vi "CountStats.vi"() -> ()   [LabVIEW 2014]
uses:
  <instrlib>/Agilent 532XX Series/Public/Configure/Configure Channel (Basic).vi
  <instrlib>/Agilent 532XX Series/Public/Configure/Configure Channel (Voltage Range).vi
  <instrlib>/Agilent 532XX Series/Public/Configure/Configure Channel (Slop).vi
  <instrlib>/Agilent 532XX Series/Public/Configure/Configure Channel (Threshold Voltage).vi
  <instrlib>/Agilent 532XX Series/Public/Configure/Measurement/Configure Measurement (Totalize Timed).vi
  <instrlib>/Agilent 532XX Series/Public/Data/Read Measurement (Statistics).vi
  <instrlib>/Agilent 532XX Series/Agilent 532XX Series.lvlib
panel:
  in  "Sample Count (1)":i32=1
  out "Standard Deviation":dbl
  out "Maximum":dbl format="%#_12g"
  out "Minimum":dbl format="%#_12g"
  out "error out":errorcluster
  out "Measurement":dbl format="%#_12g"
  in  "VISA resource name":refnum<visa-resource-name>
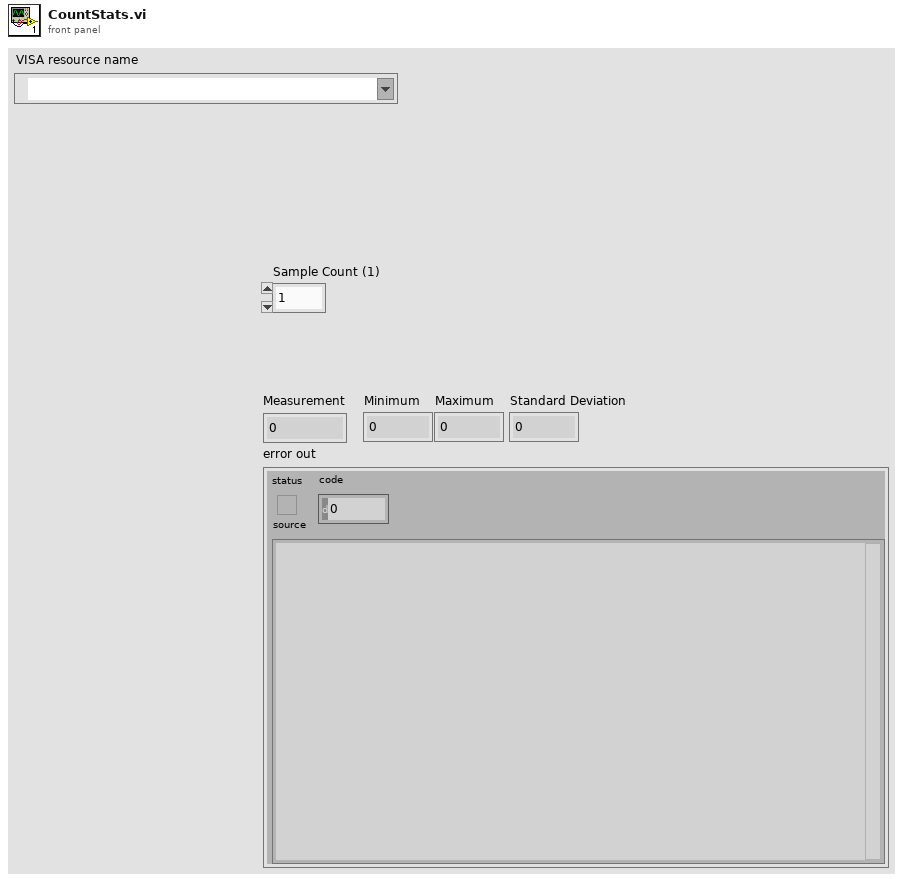
[diagram p1: front panel]
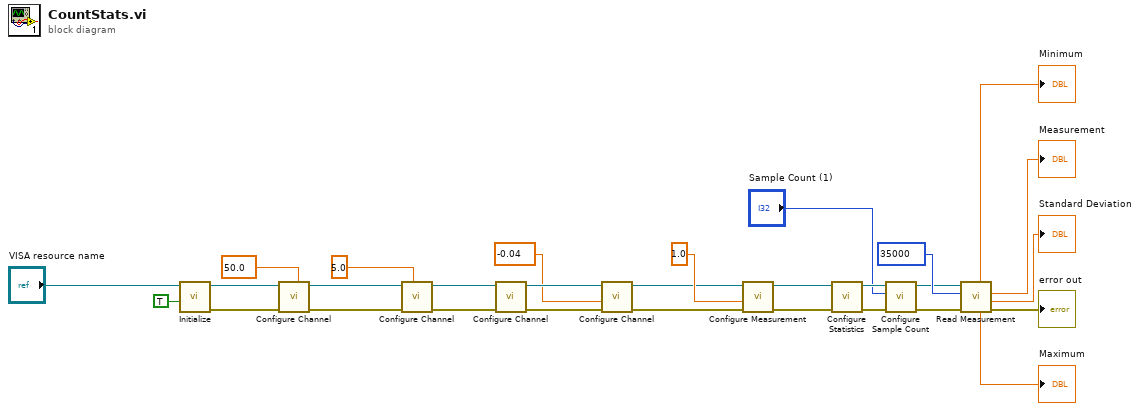
[diagram p0: block diagram]
diagram:
  w19 = 50.0 items=["50"=50.0, "1E+6"=1000000.0] ("Impedance (1E+6 Ohm)")
  n1 = call <instrlib>:"Initialize.vi"("Reset (True)"=TRUE, "VISA resource name"="VISA resource name") -> ("error out"=w21:errorcluster, "VISA resource name out"=w20:refnum<visa-resource-name>)  [unwired: 8 in]
  n2 = call-poly <instrlib>:"Configure Channel.vi"("Impedance (1E+6 Ohm)"=w19, "error in (no error)"=w21, "VISA resource name"=w20) -> ("error out"=w16:errorcluster, "VISA resource name out"=w17:refnum<visa-resource-name>)  [unwired: 7 in]
  n3 = call-poly <instrlib>:"Configure Channel.vi"("Voltage Range (5V)"=5.0, "error in (no error)"=w16, "VISA resource name"=w17) -> ("error out"=w14:errorcluster, "VISA resource name out"=w15:refnum<visa-resource-name>)  [unwired: 7 in]
  n4 = call-poly <instrlib>:"Configure Channel.vi"("error in (no error)"=w14, "VISA resource name"=w15) -> ("error out"=w13:errorcluster, "VISA resource name out"=w12:refnum<visa-resource-name>)  [unwired: 8 in]
  n5 = call-poly <instrlib>:"Configure Channel.vi"("error in (no error)"=w13, "Threshold Voltage (0 V)"=-0.04, "VISA resource name"=w12) -> ("error out"=w9:errorcluster, "VISA resource name out"=w10:refnum<visa-resource-name>)  [unwired: 7 in]
  n6 = call-poly <instrlib>:"Configure Measurement.vi"("error in (no error)"=w9, "Timed Totalize (0.1 s)"=1.0, "VISA resource name"=w10) -> ("error out"=w26:errorcluster, "VISA resource name out"=w25:refnum<visa-resource-name>)  [unwired: 7 in]
  n7 = call <instrlib>:"Configure Statistics.vi"("error in (no error)"=w26, "VISA resource name"=w25) -> ("error out"=w24:errorcluster, "VISA resource name out"=w23:refnum<visa-resource-name>)  [unwired: 8 in]
  n8 = call <instrlib>:"Configure Sample Count.vi"("error in (no error)"=w24, "Sample Count (1)"="Sample Count (1)", "VISA resource name"=w23) -> ("error out"=w1:errorcluster, "VISA resource name out"=w2:refnum<visa-resource-name>)  [unwired: 7 in]
  n9 = call-poly <instrlib>:"Read Measurement.vi"("error in (no error)"=w1, "Timeout (10000 ms)"=u32 35000, "VISA resource name"=w2) -> ("error out"=→"error out":errorcluster, "Standard Deviation"=→"Standard Deviation":dbl, "Mean"=→"Measurement":dbl, "Maximum"=→"Maximum":dbl, "Minimum"=→"Minimum":dbl)  [unwired: 3 in, 1 out]
